vi "Get Queue Status.vi"(8 "Error In":errorcluster, 11 "TDMS Log In":refnum<class "TDMS Logger.lvclass">) -> (0 "Error Out":errorcluster, 1 "# elements in queue":i32, 3 "TDMS Log Out":refnum<class "TDMS Logger.lvclass">)   [LabVIEW 2014, in "TDMS Logger.lvlib" / "TDMS Logger.lvclass"]
doc: "Use this VI to get the number of elements in the logger queue. This can be used for debugging the application and checking if the data is not passed to quickly. This VI also returns the data logger queue reference for advanced debugging and functionality.<b> DO not use this reference to enqueue data to the logger. </b>"
uses:
  TDMS Logger.lvclass
  TDMS Logger.lvclass/TDMS Logger.ctl
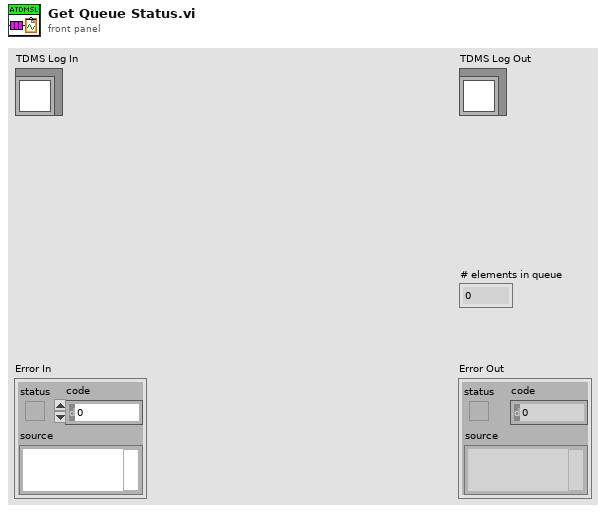
[diagram p1: front panel]
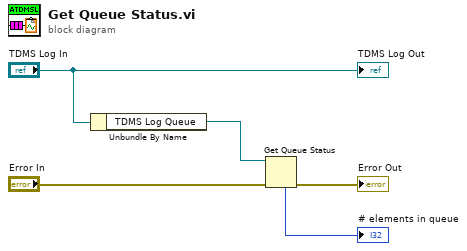
[diagram p0: block diagram]
diagram:
  n1 = Unbundle By Name("TDMS Log In") -> ("TDMS Log Queue"=w4:refnum<queue>)
  n2 = Get Queue Status(queue=w4, error in (no error)="Error In") -> (error out=→"Error Out":errorcluster, # elements in queue=→"# elements in queue":i32)  [unwired: 1 in, 6 out]
  "TDMS Log Out" <- "TDMS Log In"
